vi "a.vi"() -> ()   [LabVIEW 2021]
doc: "本VI是为《我和LabVIEW》一书编写的示例。\n关于本书的介绍请参考网页：\nhttp://ruanqizhen.spaces.live.com/blog/cns!5852D4F797C53FB6!4310.entry"
uses:
  <vilib>/sound2/lvsound2.llb/Sampling Mode.ctl
  <vilib>/sound2/lvsound2.llb/Sound Data Format.ctl
  <vilib>/measure/matone.llb/Extract Single Tone Information 1 Chan.vi
  <vilib>/measure/maspectr.llb/FFT Power Spectrum for 1 Chan.vi
  <vilib>/sound2/lvsound2.llb/Sound Input Read (DBL).vi
  <vilib>/measure/NI_MAPro.lvlib
panel:
  out "标准频率":dbl
  out "当前频率":dbl caption="检测到的频率" format="%.2p"
  out "频谱":cluster{"f0":dbl, "df":dbl, "magnitude":dbl[]}(graph)
  in  "停止":bool
  in  "选项卡控件":enum32{"弦 1", "弦 2", "弦 3", "弦 4", "弦 5", "弦 6"}(tab)
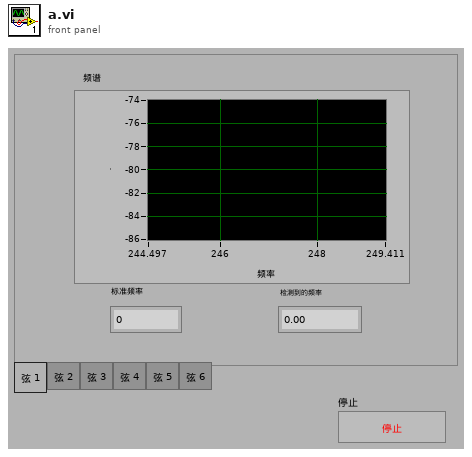
[diagram p1: front panel]
types:
  T1 = typedef "Sound Data Format.ctl" = cluster{"sample rate (S/s)":dbl, "number of channels":i32, "bits per sample":i32}
  T2 = typedef "Sampling Mode.ctl" = i32
  T3 = typedef "Sound Input Task ID.ctl" = u32
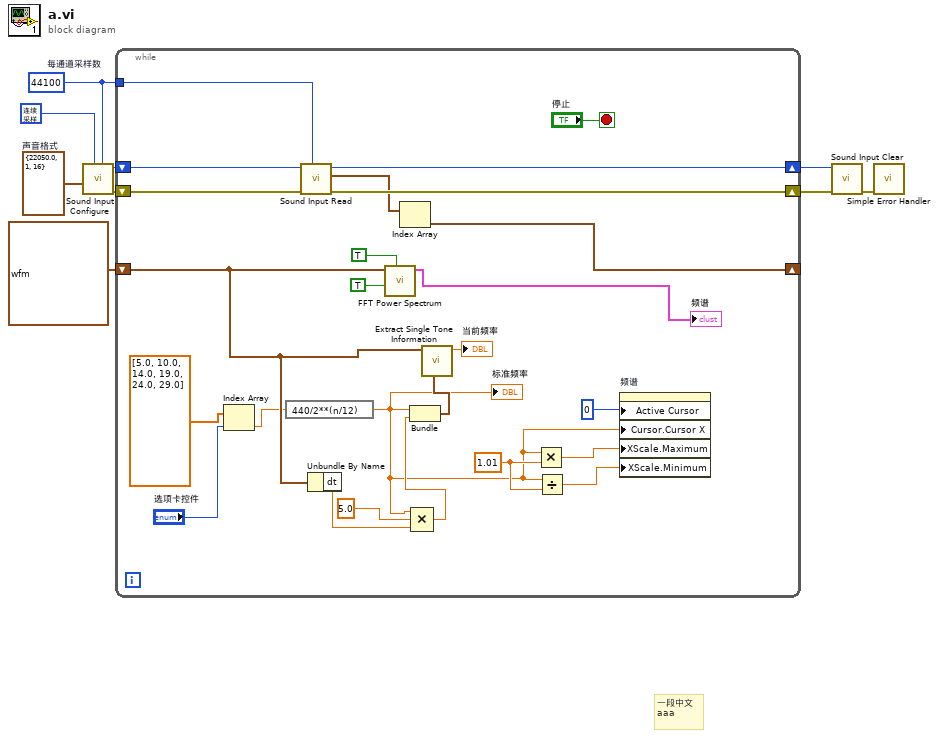
[diagram p0: block diagram]
diagram:
  w9 = T1 {"sample rate (S/s)"=22050.0, "number of channels"=1, "bits per sample"=16}  # 声音格式
  w8 = T2 1 items=["有限采样", "连续采样"] ("sample mode")
  w1 = 44100  # 每通道采样数
  # "一段中文\naaa"
  n1 = call <vilib>:"Sound Input Configure.vi"("number of samples/ch"=w1, "sample mode"=w8, "sound format"=w9) -> ("error out"=w4:errorcluster, "task ID"=w7:T3)  [unwired: 4 in, 3 out]
  n2 = while {
    shift-right: [w33] -> w5
    shift-left: w7 -> [w34]
    shift-right: [w29] -> w3
    shift-left: w4 -> [w31]
    tunnel: w1 -> [w30]
    shift-right: [w27] -> _
    shift-left: waveform(dbl) {"t0"=timestamp(0 s since 1904-01-01), "dt"=1.0, "Y"=[]} ("Data") -> [w25]
    stop <- "停止" stop-if-true
    w18 = 1.01 ("y")
    n3 = Index Array(array=dbl[] [5.0, 10.0, 14.0, 19.0, 24.0, 29.0], index="选项卡控件") -> (element=w10:dbl)
    n4 = expression code="440/2**(n/12)"(w10) -> (w14:dbl)
    "标准频率" <- w14
    n5 = call-poly <vilib>:"Sound Input Read.vi"("number of samples/ch"=w30, "error in (no error)"=w31, "task ID"=w34) -> ("error out"=w29:errorcluster, "data"=w28:waveform(dbl)[], "task ID out"=w33:T3)  [unwired: 1 in, 5 out]
    n6 = Unbundle By Name(w25) -> ("dt"=w21:dbl)
    n7 = call-poly <vilib>:"FFT Power Spectrum.vi"("restart averaging (F)"=TRUE, "dB On (F)"=TRUE, "time signal"=w25) -> ("power spectrum"=→"频谱":cluster{"f0":dbl, "df":dbl, "magnitude":dbl[]})  [unwired: 3 in, 5 out]
    n8 = Index Array(array=w28) -> (element=w27:waveform(dbl))  [unwired: 1 in]
    n9 = Compound Arithmetic op=MULTIPLY(w14, 5.0 ("search (+/- % of Fsampl.)"), w21) -> (w19:dbl)
    n10 = Bundle(w14, w19) -> (w22:cluster{dbl, dbl})  [unwired: 1 out]
    n11 = call-poly <vilib>:"Extract Single Tone Information.vi"("advanced search"=w22, "time signal in"=w25) -> ("detected frequency"=→"当前频率":dbl)  [unwired: 2 in, 7 out]
    n12 = Multiply(x=w14, y=w18) -> (x*y=w17:dbl)
    n13 = Divide(x=w14, y=w18) -> (x/y=w16:dbl)
    n14 = property on="频谱" class="WFGraph (strict)"("Active Cursor"=u32 0 ("活动游标"), "Cursor.Cursor X"=w14, "XScale.Maximum"=w17, "XScale.Minimum"=w16) -> ()  [unwired: 2 in, 2 out]
  }
  n15 = call <vilib>:"Sound Input Clear.vi"("error in (no error)"=w3, "task ID"=w5) -> ("error out"=w6:errorcluster)  [unwired: 9 out]
  n16 = call <vilib>:"Simple Error Handler.vi"("error in (no error)"=w6) -> ()  [unwired: 1 in, 8 out]
